vi "VI-Move Wire Bend.vi"(0 "Terminal in":refnum<vi>, 9 "Horizontal":i16=350, 11 "error in (no error)":errorcluster) -> (15 "error out":errorcluster)   [LabVIEW 2015]
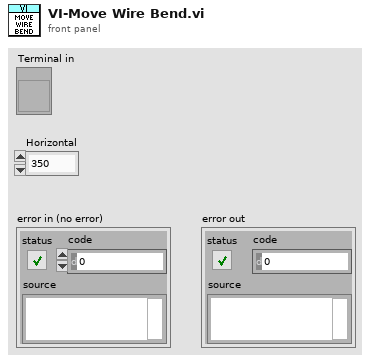
[diagram p1: front panel]
types:
  T1 = cluster{"Position":cluster{"h":i16, "v":i16}, "Flags":i32, "Type":enum32{"LooseEnd", "Endpoint", "Bend", "Junction"}, "Up Joint Index":i16, "Down Joint Index":i16, "Left Joint Index":i16, "Right Joint Index":i16}[]
  T2 = enum32{"LooseEnd", "Endpoint", "Bend", "Junction"}
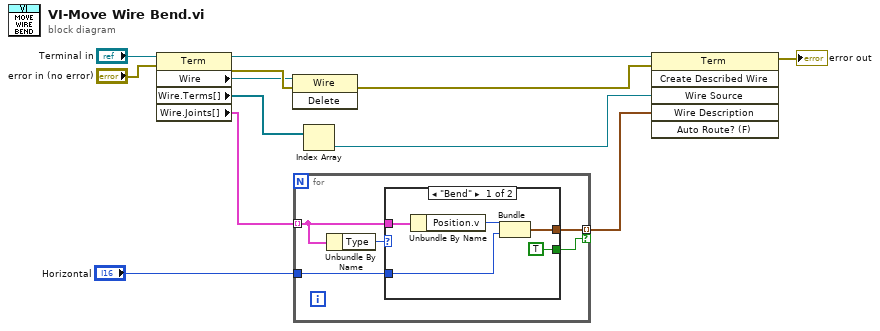
[diagram p0: block diagram]
diagram:
  n1 = property class="Term"(reference="Terminal in", error in="error in (no error)") -> (reference out=w10:refnum<vi>, error out=w6:errorcluster, "Wire"=w5:refnum<vi>, "Wire.Terms[]"=w3:refnum<vi>[], "Wire.Joints[]"=w7:T1)
  n2 = invoke class="Wire" method="Delete"(reference=w5, error in=w6) -> (error out=w12:errorcluster)  [unwired: 1 in, 2 out]
  n3 = for {
    tunnel: w7 -> [w14] mode=indexing
    tunnel: [w16] -> w1 mode=indexing if=w15
    tunnel: "Horizontal" -> [w13]
    n4 = Unbundle By Name(w14) -> ("Type"=w17:T2)
    n5 = case shown="\"Bend\"" w17 {
      tunnel: [w20 _] -> w16
      tunnel: [TRUE _] -> w15
      tunnel: w14 -> [w19 _]
      tunnel: w13 -> [w18 _]
      frame "Bend" {
        n6 = Unbundle By Name(w19) -> ("Position.v"=w21:i16)
        n7 = Bundle("v"=w21, "Horizontal"=w18) -> (w20:cluster{"v":i16, "Horizontal":i16})  [unwired: 1 in]
      }
      frame "Endpoint", Default {
      }
    }
  }
  n8 = Index Array(array=w3) -> (element=w2:refnum<vi>)  [unwired: 1 in]
  n9 = invoke class="Term" method="Create Described Wire"(reference=w10, error in=w12, "Wire Source"=w2, "Wire Description"=w1) -> (error out=→"error out":errorcluster)  [unwired: 2 in, 5 out]
